vi "15_ВПГрафикФункции.vi"() -> ()   [LabVIEW 2016]
panel:
  out "Waveform Graph":dynamicdata(graph)
  in  "Numeric":dbl
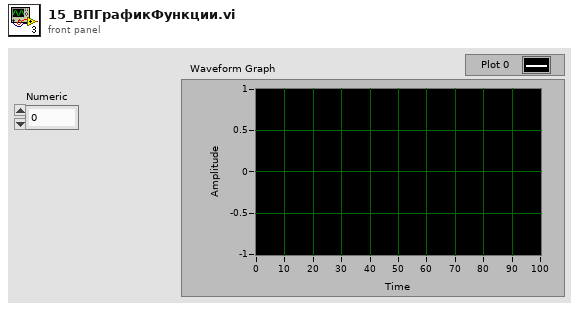
[diagram p1: front panel]
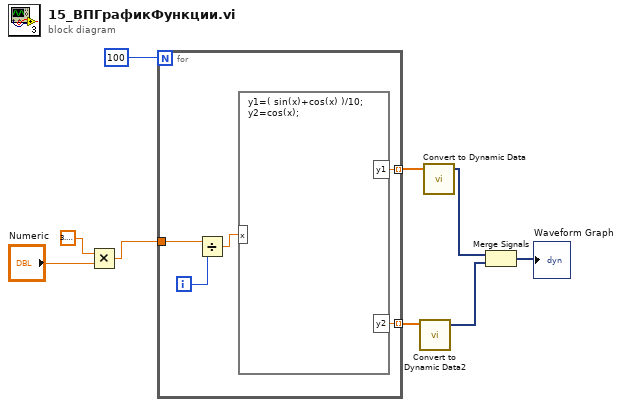
[diagram p0: block diagram]
diagram:
  n1 = Multiply(x=3.141592653589793, y="Numeric") -> (x*y=w6:dbl)
  n2 = for {
    N: 100 -> [_]
    tunnel: w6 -> [w13]
    tunnel: [w11] -> w4 mode=indexing
    tunnel: [w10] -> w1 mode=indexing
    i -> [w14]
    n3 = Divide(x=w13, y=w14) -> (x/y=w12:dbl)
    n4 = formula code="y1=( sin(x)+cos(x) )/10;\ny2=cos(x);"("x"=w12) -> ("y1"=w10:dbl, "y2"=w11:dbl)
  }
  n5 = call "Convert to Dynamic Data2"("Array"=w4) -> ("Dynamic Data Type"=w2:dynamicdata)  [unwired: 3 in]
  n6 = call "Convert to Dynamic Data"("Array"=w1) -> ("Dynamic Data Type"=w3:dynamicdata)  [unwired: 3 in]
  n7 = Merge Signals(w3, w2) -> (→"Waveform Graph":dynamicdata)
